vi "gentec-M-Link.Set Waveform Averages.vi"(0 "VISA resource In":refnum<visa-resource-name>, 2 "Waveform Averages":T1 items=["None", "2", "4", "8", "16", "32", "64", "128"], 5 "error in (no error)":errorcluster) -> (11 "Data Read":string, 13 "Read Timeout":bool, 14 "VISA resource Out":refnum<visa-resource-name>, 16 "Success":bool, 19 "error out":errorcluster)   [LabVIEW 2014, in "gentec-M-Link - Driver.lvlib"]
doc: "Data to write: avg<n> where n is a number; valid are values from 1 to 8\n\nSets the sampling size of noise suppression. Valid averages are powers of 2 from 1 to 128. If a non valid argument is sent, Err is returned and the value is left unchanged."
uses:
  gentec-M-Link - Driver.lvlib
  Type Defs/gentec-M-Link.Waveform Averages.ctl
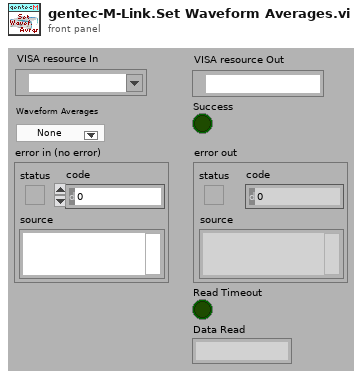
[diagram p1: front panel]
types:
  T1 = typedef "gentec-M-Link - Driver.lvlib/gentec-M-Link.Waveform Averages.ctl" = u16
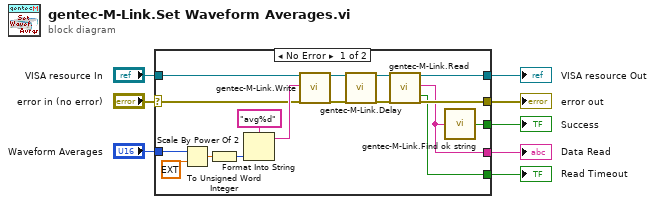
[diagram p0: block diagram]
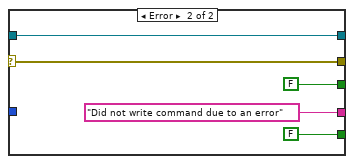
[diagram p2: hidden frame]
diagram:
  n1 = case shown="No Error" "error in (no error)" {
    selector: "error in (no error)" -> [w18 w30]
    tunnel: [w23 w30] -> w7
    tunnel: "VISA resource In" -> [w21 w29]
    tunnel: [w20 FALSE ("Found")] -> w5
    tunnel: [w19 w29] -> w4
    tunnel: "Waveform Averages" -> [w17 _]
    tunnel: [w10 "Did not write command due to an error" ("Data Read")] -> w2
    tunnel: [w9 FALSE ("Read Timeout")] -> w1
    frame No Error {
      n2 = Scale By Power Of 2(n=w17, x=ext 1.0) -> (x*2^n=w16:ext)
      n3 = To Unsigned Word Integer(number=w16) -> (unsigned 16bit integer=w15:u16)
      n4 = Format Into String(format string="avg%d", w15) -> (resulting string=w24:string)  [unwired: 2 in, 1 out]
      n5 = call "gentec-M-Link.Write.vi"("VISA resource (In)"=w21, "Data To Write"=w24, "error in (no error)"=w18) -> ("VISA resource (Out)"=w12:refnum<visa-resource-name>, "error out"=w22:errorcluster)  [unwired: 14 in, 1 out]
      n6 = call "gentec-M-Link.Delay.vi"("VISA resource In"=w12, "error in (no error)"=w22) -> ("VISA resource Out"=w11:refnum<visa-resource-name>, "error out"=w13:errorcluster)  [unwired: 16 in]
      n7 = call "gentec-M-Link.Read.vi"("VISA resource (In)"=w11, "error in (no error)"=w13) -> ("VISA resource (Out)"=w19:refnum<visa-resource-name>, "Data Read"=w10:string, "Read Timeout"=w9:bool, "error out"=w23:errorcluster)  [unwired: 13 in, 1 out]
      n8 = call "gentec-M-Link.Find ok string.vi"("string"=w10) -> ("Found"=w20:bool)
    }
    frame Error {
    }
  }
  "error out" <- w7
  "Success" <- w5
  "VISA resource Out" <- w4
  "Data Read" <- w2
  "Read Timeout" <- w1
